vi "Muliti_XY_dispense.vi"(0 "Vacuum Setting (0000)":i64=20, 1 "Pressure":i16=20, 6 "Path count":i32, 8 "Speed":dbl=20.0 format="%#_13g", 9 "distances":dbl[][](array[numeric]), 10 "Ultimus V in":refnum<class "Ultimus V2.lvclass">, 11 "Motion in":refnum<class "Motion.lvclass">) -> (2 "Ultimus V out":refnum<class "Ultimus V2.lvclass">, 3 "Motion out":refnum<class "Motion.lvclass">)   [LabVIEW 2016]
uses:
  Classes/Controllers/Motion/Copy of Motion Folder/Motion.lvclass
  Classes/Controllers/Dispenser/Copy of Ultimus V2 Folder/Ultimus V2.lvclass
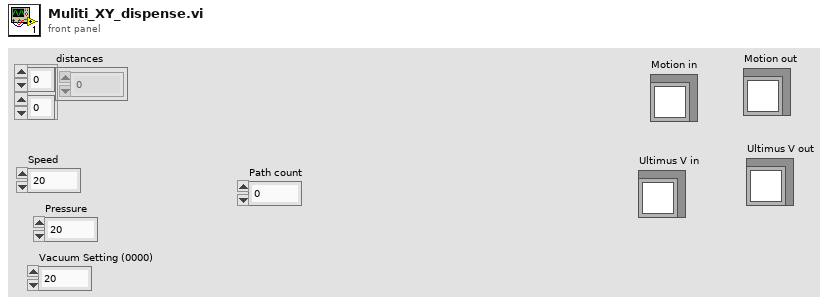
[diagram p1: front panel]
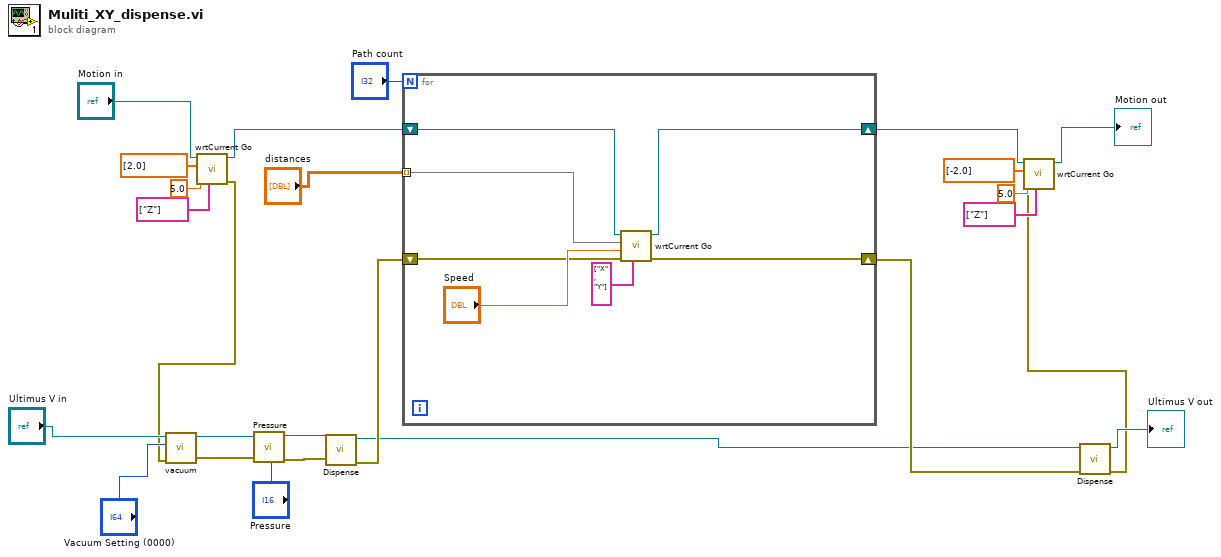
[diagram p0: block diagram]
diagram:
  n1 = call-dynamic "wrtCurrent Go.vi"("axis names"=string[] ["Z"], "Speed"=5.0, "distances"=dbl[] [2.0], "Motion in"="Motion in") -> ("error out"=w1:errorcluster, "Motion out"=w8:refnum<class "Motion.lvclass">)  [unwired: 6 in]
  n2 = call "vacuum.vi"("error in (no error)"=w1, "Vacuum Setting (0000)"="Vacuum Setting (0000)", "Ultimus V in"="Ultimus V in") -> ("error out"=w21:errorcluster, "Ultimus V out"=w24:refnum<class "Ultimus V2.lvclass">)  [unwired: 7 in]
  n3 = call-dynamic "Pressure.vi"("error in (no error)"=w21, "Pressure"="Pressure", "Ultimus V in"=w24) -> ("error out"=w20:errorcluster, "Ultimus V out"=w25:refnum<class "Ultimus V2.lvclass">)  [unwired: 7 in]
  n4 = call-dynamic "Dispense.vi"("error in (no error)"=w20, "Ultimus V in"=w25) -> ("error out"=w19:errorcluster, "Ultimus V out"=w17:refnum<class "Ultimus V2.lvclass">)  [unwired: 8 in]
  n5 = for {
    N: "Path count" -> [_]
    shift-right: [w30] -> w18
    shift-left: w19 -> [w31]
    shift-right: [w28] -> w4
    shift-left: w8 -> [w29]
    tunnel: "distances" -> [w27] mode=indexing
    n6 = call-dynamic "wrtCurrent Go.vi"("axis names"=string[] ["X", "Y"], "error in (no error)"=w31, "Speed"="Speed", "distances"=w27, "Motion in"=w29) -> ("error out"=w30:errorcluster, "Motion out"=w28:refnum<class "Motion.lvclass">)  [unwired: 5 in]
  }
  n7 = call-dynamic "Dispense.vi"("error in (no error)"=w18, "Ultimus V in"=w17) -> ("error out"=w2:errorcluster, "Ultimus V out"=→"Ultimus V out":refnum<class "Ultimus V2.lvclass">)  [unwired: 8 in]
  n8 = call-dynamic "wrtCurrent Go.vi"("axis names"=string[] ["Z"], "error in (no error)"=w2, "Speed"=5.0, "distances"=dbl[] [-2.0], "Motion in"=w4) -> ("Motion out"=→"Motion out":refnum<class "Motion.lvclass">)  [unwired: 5 in, 1 out]
